vi "Calc All Texture Deltas.vi"(10 "Texture":T6, 11 "Sorted Triangle":T1={"Top Vertex"={"Position"={"x"=0.0, "y"=0.0, "z"=0.0}, "UV"={"u"=0.0, "v"=0.0}, "Colour"=12517256}, "Mid Vertex"={"Position"={"x"=0.0, "y"=0.0, "z"=0.0}, "UV"={"u"=0.0, "v"=0.0}, "Colour"=12517256}, "Bottom Vertex"={"Position"={"x"=0.0, "y"=0.0, "z"=0.0}, "UV"={"u"=0.0, "v"=0.0}, "Colour"=12517256}, "Alpha"=0.0, "Alpha Blending Enabled"=FALSE, "Colour"=0, "Material"={"Diffuse Colour"=0, "Texture"={"Pixels"=refnum, "Size"={"Width"=0, "Height"=0}}}} {"Bottom Vertex"."UV"."v" min=0 max=1 step=0.1; "Bottom Vertex"."UV"."u" min=0 max=1 step=0.1; "Mid Vertex"."UV"."v" min=0 max=1 step=0.1; "Mid Vertex"."UV"."u" min=0 max=1 step=0.1; "Top Vertex"."UV"."v" min=0 max=1 step=0.1; "Top Vertex"."UV"."u" min=0 max=1 step=0.1}) -> (3 "Texels Step Deltas":T8)   [LabVIEW 2020, in "Raster (FPGA).lvlib"]
uses:
  Raster (FPGA).lvlib
  Texel Step Deltas (BMT).ctl
  Point 2D (SGL).ctl
  Texture.ctl
  Rectangle Dimensions.ctl
  3D/Triangle (Sorted).ctl
  3D/Vertex.ctl
  3D/Vector 3D.ctl
  UV.ctl
  3D/Material.ctl
  3D/3D (FPGA).lvlib
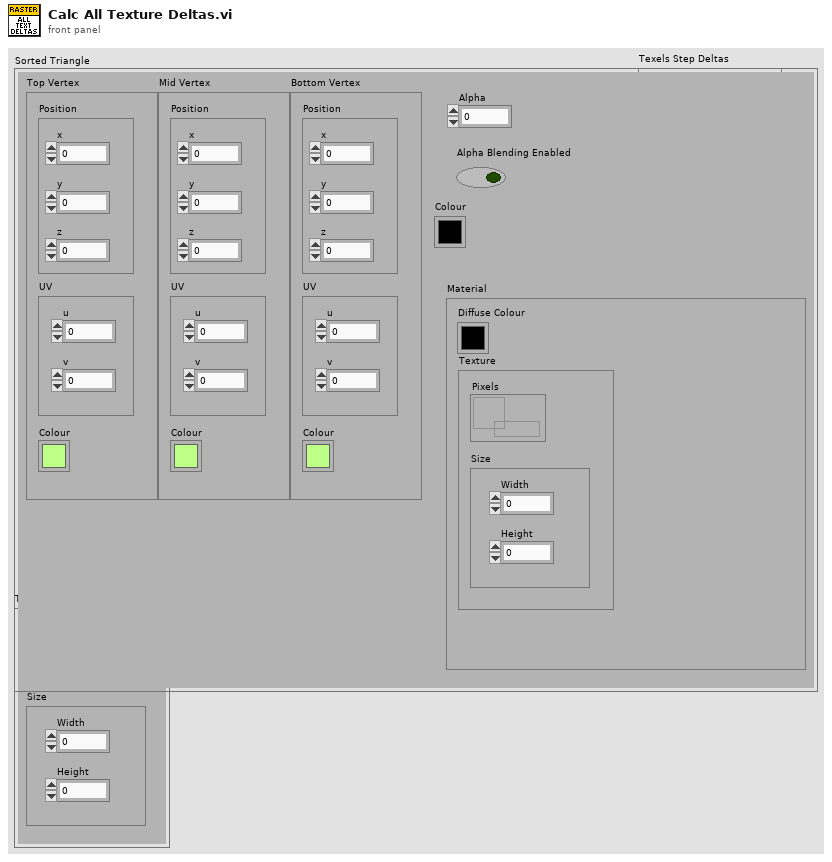
[diagram p1: front panel]
types:
  T1 = typedef "3D (FPGA).lvlib/Triangle (Sorted).ctl" = cluster{"Top Vertex":T2, "Mid Vertex":T2, "Bottom Vertex":T2, "Alpha":dbl, "Alpha Blending Enabled":bool, "Colour":u32, "Material":T5}
  T2 = typedef "3D (FPGA).lvlib/Vertex.ctl" = cluster{"Position":T3, "UV":T4, "Colour":u32}
  T3 = typedef "3D (FPGA).lvlib/Vector 3D.ctl" = cluster{"x":sgl, "y":sgl, "z":sgl}
  T4 = typedef "Raster (FPGA).lvlib/UV.ctl" = cluster{"u":sgl, "v":sgl}
  T5 = typedef "3D (FPGA).lvlib/Material.ctl" = cluster{"Diffuse Colour":u32, "Texture":T6}
  T6 = typedef "Raster (FPGA).lvlib/Texture.ctl" = cluster{"Pixels":refnum<data-value>, "Size":T7}
  T7 = typedef "Raster (FPGA).lvlib/Rectangle Dimensions.ctl" = cluster{"Width":u32, "Height":u32}
  T8 = typedef "Raster (FPGA).lvlib/Texel Step Deltas (BMT).ctl" = cluster{"Bottom To Top":T9, "Bottom To Middle":T9, "Middle To Top":T9}
  T9 = typedef "Raster (FPGA).lvlib/Point 2D (SGL).ctl" = cluster{"x":sgl, "y":sgl}
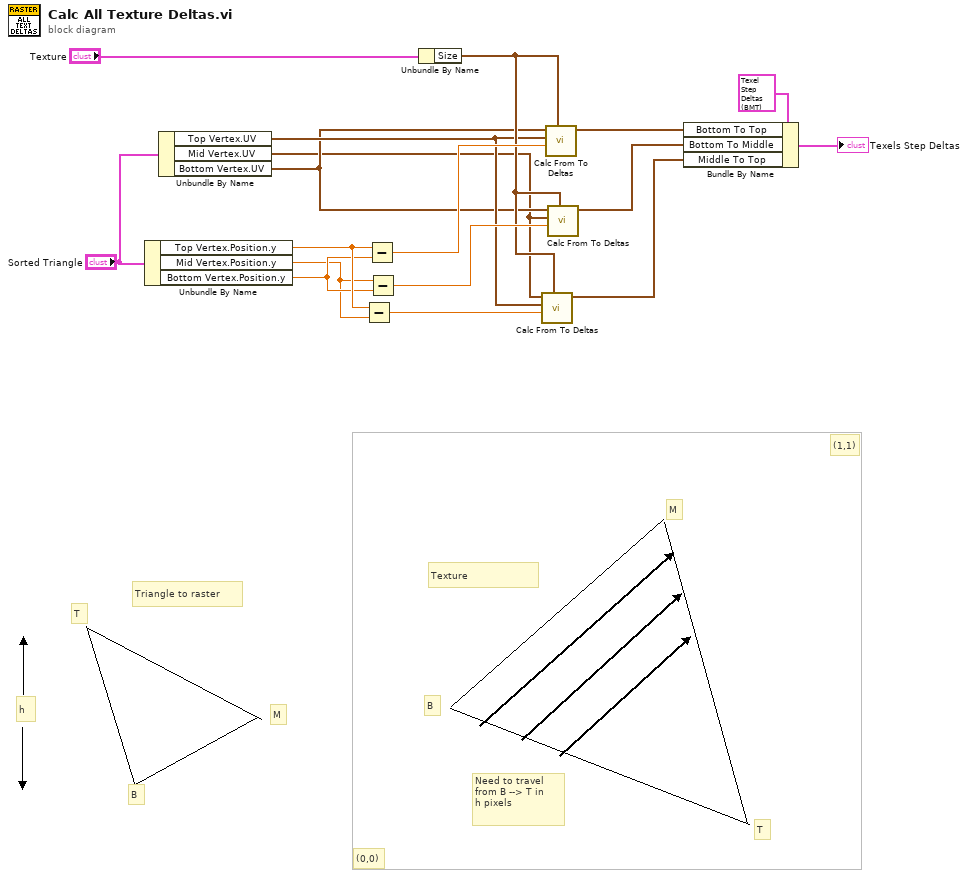
[diagram p0: block diagram]
diagram:
  # "(0,0)"
  # "(1,1)"
  # "h"
  # "Texture"
  # "Triangle to raster"
  # "M"
  # "T"
  # "B"
  # "Need to travel from B --> T in \nh pixels"
  # "T"
  # "M"
  # "B"
  n1 = Unbundle By Name("Sorted Triangle") -> ("Top Vertex.Position.y"=w3:sgl, "Mid Vertex.Position.y"=w1:sgl, "Bottom Vertex.Position.y"=w2:sgl)
  n2 = Unbundle By Name("Sorted Triangle") -> ("Top Vertex.UV"=w6:T4, "Mid Vertex.UV"=w4:T4, "Bottom Vertex.UV"=w5:T4)
  n3 = Subtract(x=w3, y=w1) -> (x-y=w15:sgl)
  n4 = Subtract(x=w3, y=w2) -> (x-y=w17:sgl)
  n5 = Subtract(x=w1, y=w2) -> (x-y=w16:sgl)
  n6 = Unbundle By Name("Texture") -> ("Size"=w8:T7)
  n7 = call "Calc From To Deltas.vi"("Texture Dimensions"=w8, "Steps"=w15, "To"=w6, "From"=w4) -> ("Deltas (Texels Per Step)"=w10:T4)  [unwired: 7 in]
  n8 = call "Calc From To Deltas.vi"("Texture Dimensions"=w8, "Steps"=w17, "To"=w6, "From"=w5) -> ("Deltas (Texels Per Step)"=w12:T4)  [unwired: 7 in]
  n9 = call "Calc From To Deltas.vi"("Texture Dimensions"=w8, "Steps"=w16, "To"=w4, "From"=w5) -> ("Deltas (Texels Per Step)"=w11:T4)  [unwired: 7 in]
  n10 = Bundle By Name(cluster=T8 {"Bottom To Top"={"x"=0.0, "y"=0.0}, "Bottom To Middle"={"x"=0.0, "y"=0.0}, "Middle To Top"={"x"=0.0, "y"=0.0}} ("Texels Step Deltas"), "Bottom To Top"=w12, "Bottom To Middle"=w11, "Middle To Top"=w10) -> (→"Texels Step Deltas":T8)
